vi "FROG.vi"(9 "data":dbl[][](array[numeric]), 10 "wl":dbl[](array[numeric]), 11 "time":dbl[](array[numeric])) -> ()   [LabVIEW 2019]
panel:
  out "XY Graph":cluster{dbl[], "time":dbl[]}(graph)
  out "XY Graph 2":cluster{dbl[], dbl[]}(graph)
  out "element 2":i32
  out "x-y":i32
  out "element":i32
  out "Intensity Graph":dbl[][](graph)
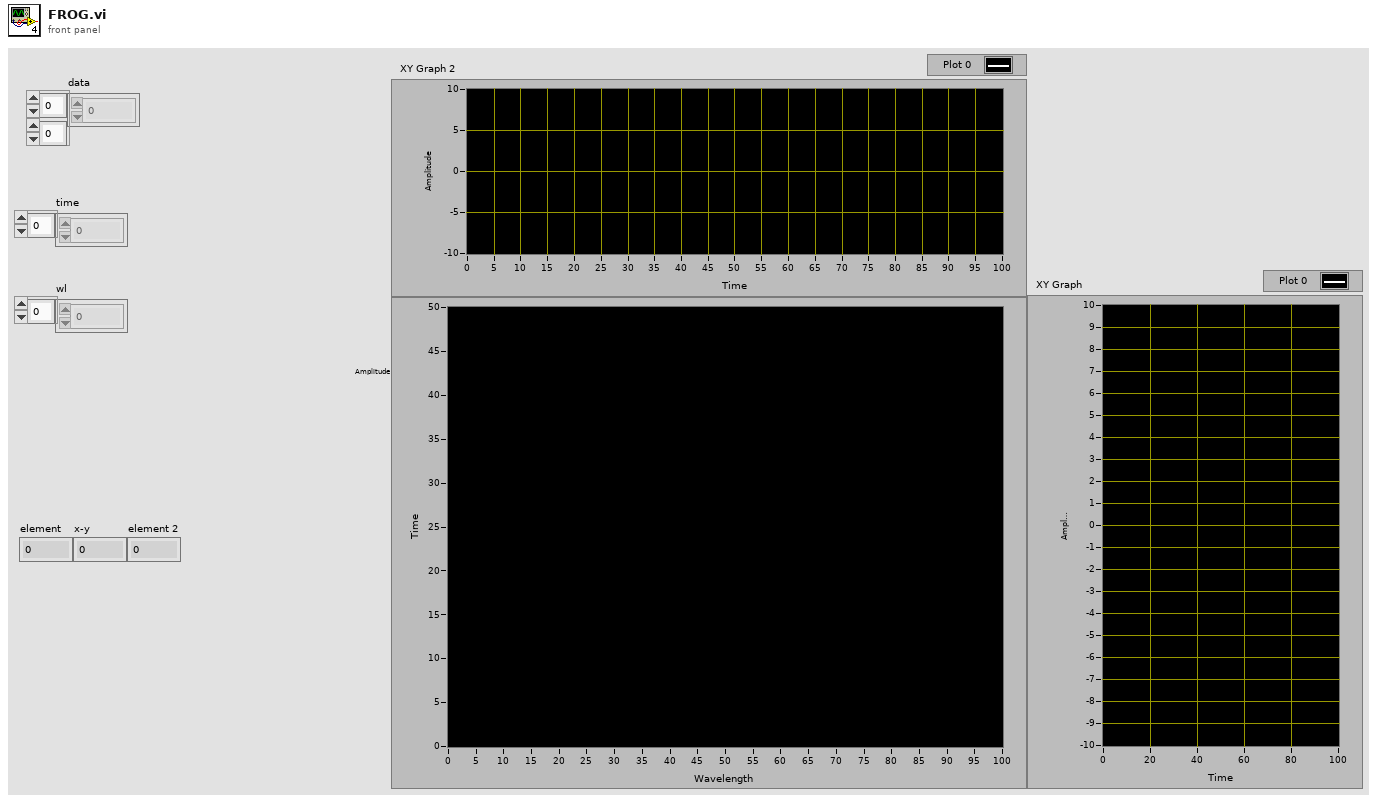
[diagram p1: front panel]
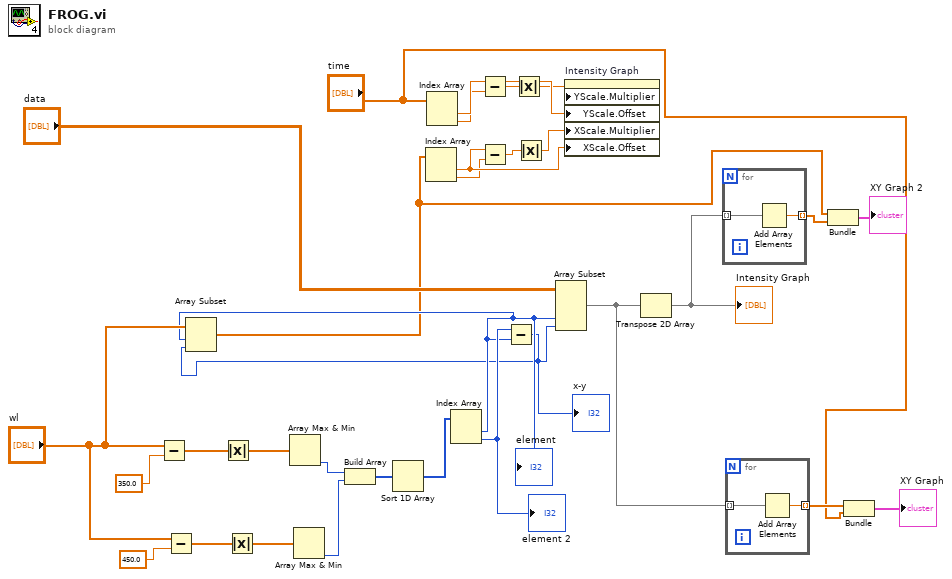
[diagram p0: block diagram]
diagram:
  n1 = Subtract(x="wl", y=350.0) -> (x-y=w30:dbl[])
  n2 = Subtract(x="wl", y=450.0) -> (x-y=w27:dbl[])
  n3 = Absolute Value(x=w30) -> (abs(x)=w29:dbl[])
  n4 = Absolute Value(x=w27) -> (abs(x)=w26:dbl[])
  n5 = Array Max & Min(array=w29) -> (min index (indices)=w24:i32)  [unwired: 3 out]
  n6 = Array Max & Min(array=w26) -> (min index (indices)=w23:i32)  [unwired: 3 out]
  n7 = Build Array(w24, w23) -> (w22:i32[])
  n8 = Sort 1D Array(array=w22) -> (sorted array=w21:i32[])
  n9 = Index Array(array="time") -> (element #1=w19:dbl, element #2=w18:dbl)  [unwired: 2 in]
  n10 = Index Array(array=w21) -> (element #1=w14:i32, element #2=w20:i32)  [unwired: 2 in]
  "element" <- w14
  "element 2" <- w20
  n11 = Subtract(x=w19, y=w18) -> (x-y=w17:dbl)
  n12 = Subtract(x=w20, y=w14) -> (x-y=w13:i32)
  "x-y" <- w13
  n13 = Array Subset(array="wl", index=w14, length=w13) -> (w2:dbl[])
  n14 = Index Array(array=w2) -> (element #1=w12:dbl, element #2=w11:dbl)  [unwired: 2 in]
  n15 = Subtract(x=w12, y=w11) -> (x-y=w10:dbl)
  n16 = Absolute Value(x=w17) -> (abs(x)=w16:dbl)
  n17 = Absolute Value(x=w10) -> (abs(x)=w9:dbl)
  n18 = Array Subset(array="data", index (col)=w14, length (col)=w13) -> (w7:dbl[][])  [unwired: 2 in]
  n19 = property on="Intensity Graph" class="IntGraph (strict)"("YScale.Multiplier"=w16, "YScale.Offset"=w19, "XScale.Multiplier"=w9, "XScale.Offset"=w12) -> ()  [unwired: 2 in, 2 out]
  n20 = Transpose 2D Array(2D array=w7) -> (transposed array=w8:dbl[][])
  "Intensity Graph" <- w8
  n21 = for {
    tunnel: w8 -> [w33] mode=indexing
    tunnel: [w32] -> w3 mode=indexing
    n22 = Add Array Elements(numeric array=w33) -> (sum=w32:dbl)
  }
  n23 = for {
    tunnel: w7 -> [w35] mode=indexing
    tunnel: [w34] -> w6 mode=indexing
    n24 = Add Array Elements(numeric array=w35) -> (sum=w34:dbl)
  }
  n25 = Bundle(w2, w3) -> (→"XY Graph 2":cluster{dbl[], dbl[]})  [unwired: 1 in]
  n26 = Bundle(w6, "time"="time") -> (→"XY Graph":cluster{dbl[], "time":dbl[]})  [unwired: 1 in]
